vi "运维调试_氨氮.vi"() -> ()   [LabVIEW 2016, in "斯坦道氨氮.lvlib"]
uses:
  <vilib>/Utility/miscctls.llb/LVPointTypeDef.ctl
  <vilib>/Utility/config.llb/NI_LVConfig.lvlib
  <vilib>/ptbypt/NI_PtbyPt.lvlib
panel:
  in  "仪器参数设置":bool
  in  "模块启用":bool
  in  "串口设置":bool
  in  "备用系数一键写入":bool
  in  "公式一键写入":bool
  in  "流程路径":path=path "C:/Users/STD/Documents/斯坦道流程文件/流程.xml"
  in  "曲线模型":cluster{"X^2":dbl, "X":dbl, "B":dbl, "r^2":dbl}(xcontrol)
  out "字符串":string
  in  "质控参数设置":bool
  in  "自动测试量程配置":T1
  out "温度2":sgl
  out "温度1":sgl
  out "ADC":sgl
  out "固件版本号":string
  in  "数组":string[](array[string])
  in  "备用系数写入":bool
  in  "备用系数读取":bool
  in  "备用系数":T2
  in  "量程切换阈值写入":bool
  in  "量程切换阈值读取":bool
  in  "量程切换阈值":cluster{"阈值":dbl, "标液浓度":dbl}
  in  "参数下拉列表":enum16{"总磷", "总氮", "氨氮"}(ring)=enum."氨氮"
  in  "量程下拉列表":enum16{"低量程", "高量程"}(ring)
  in  "测量模式下拉列表":enum16{"水样测量", "零点核查", "跨度核查", "标样核查", "加标回收"}(ring)
  in  "公式":cluster{"X^2":dbl, "X":dbl, "b":dbl}
  in  "写公式":bool
  in  "读公式":bool
  in  "返回":bool
  in  "设置":bool
  out "序列号":string="序列号"
  out "测量数据":T3(xcontrol)
  out "集成报警信息":string
  out "定时启动":bool
  out "运行状态":T4(xcontrol)
  in  "停止":bool
  in  "手动启动":bool
  in  "单步测试":bool
  in  "总磷氨氮调试":u16[](xcontrol)
  out "F3":sgl format="%#.6f"
  out "F2":sgl format="%#.6f"
  out "F1":sgl format="%#.6f"
  out "F0":sgl format="%#.6f"
  out "多列列表框":i32(listbox)
  # "参数设置"
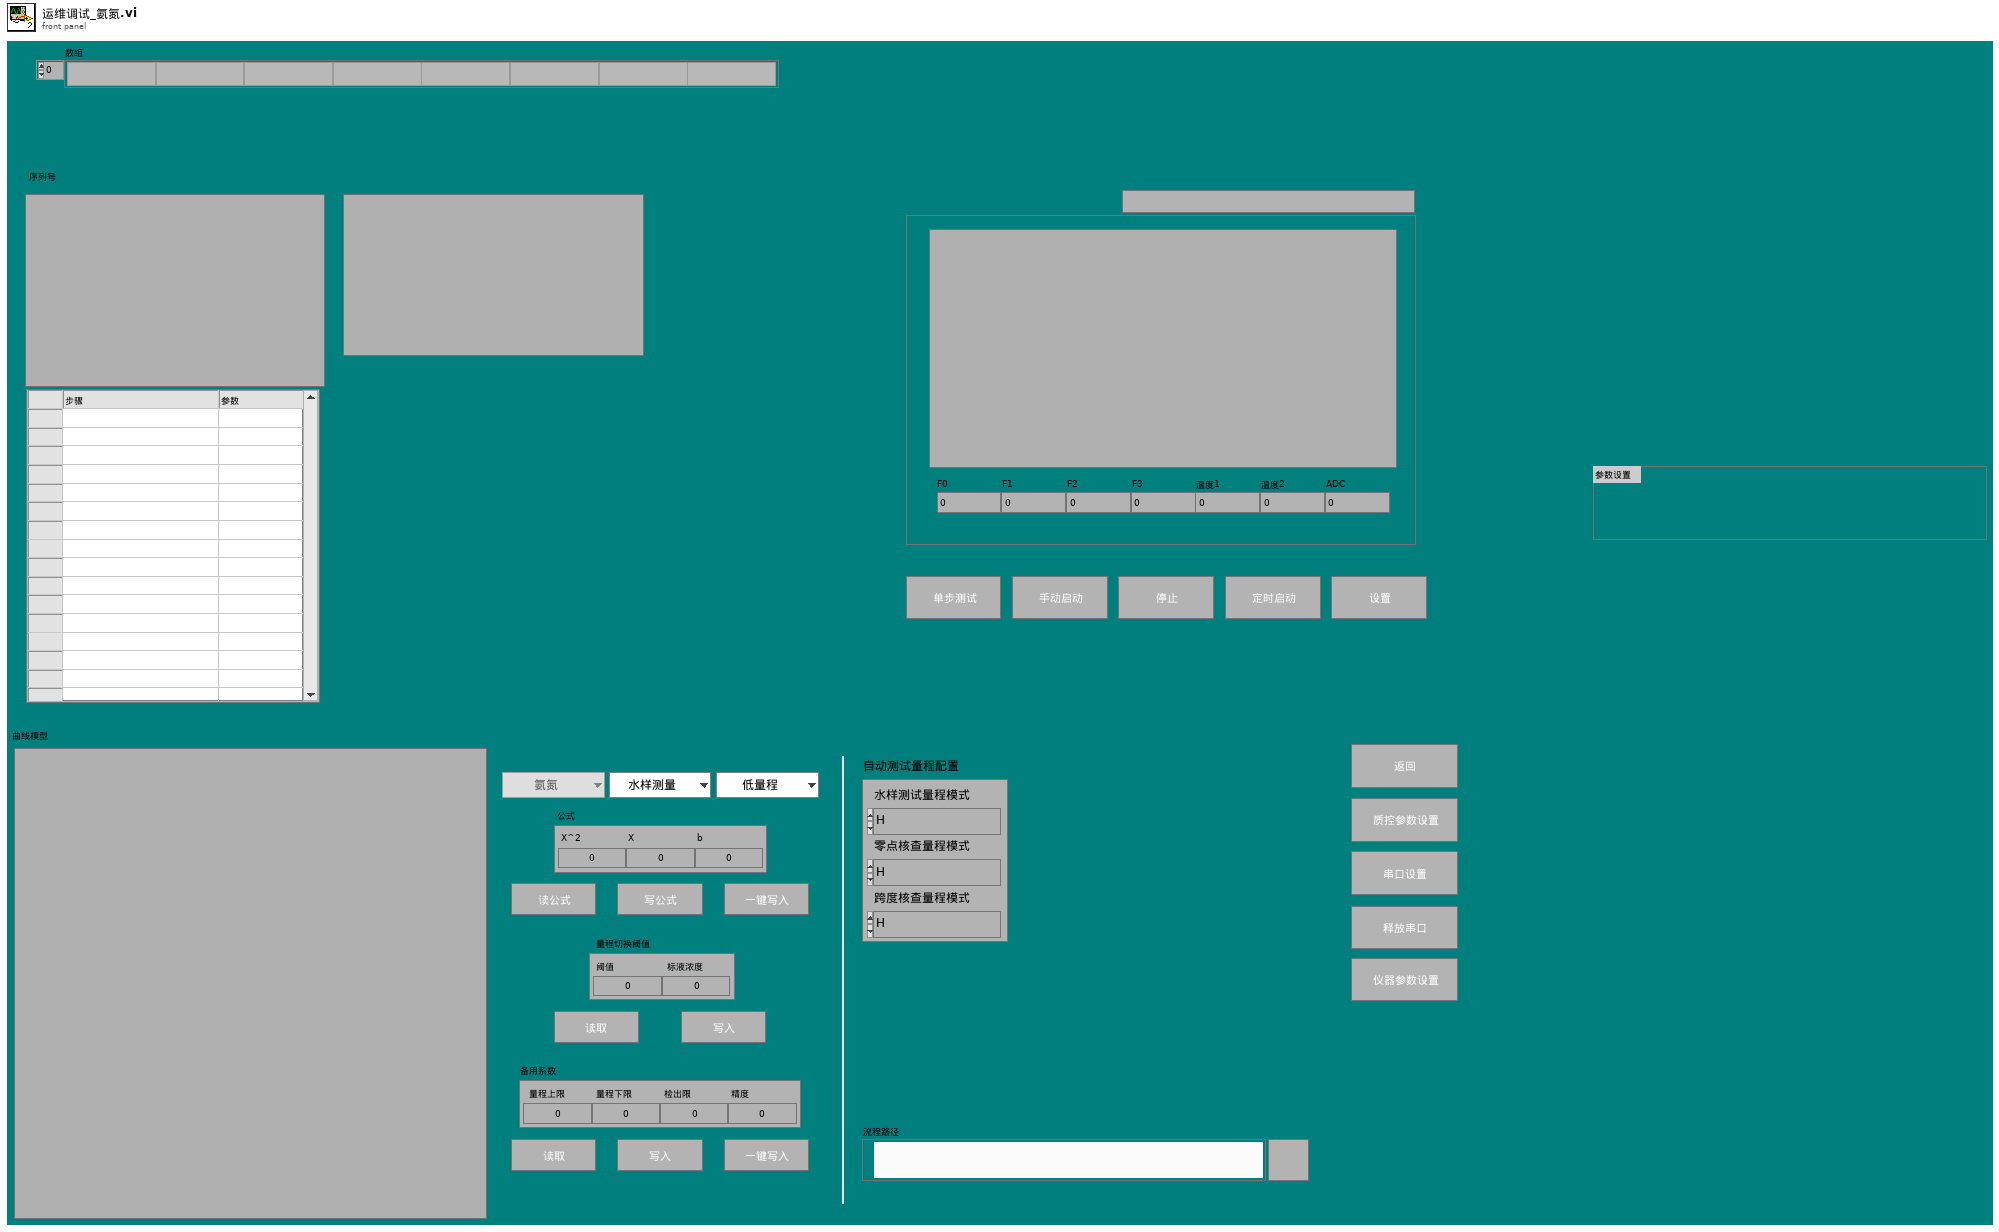
[diagram p1: front panel]
types:
  T1 = cluster{"水样测试量程模式":enum16{"H", "L", "AUTO"}, "空白核查量程模式":enum16{"H", "L", "AUTO"}, "跨度核查量程模式":enum16{"H", "L", "AUTO"}}
  T2 = cluster{"量程上限":dbl, "量程下限":dbl, "检出限":dbl, "精度":dbl}
  T3 = cluster{"flowid":u16, "测量精度":u16, "测量数据区":cluster{"因子编码":u32, "单位":u16, "标样参考值":sgl, "水样数据时间":timestamp, "水样实测值":sgl, "水样数据标识":string, "标样数据时间":timestamp, "标样实测值":sgl, "标样数据标识":string, "空白数据时间":timestamp, "空白实测值":sgl, "空白数据标识":string, "零点核查数据时间":timestamp, "零点核查实测值":sgl, "零点核查数据标识":string, "跨度核查数据时间":timestamp, "跨度核查实测值":sgl, "跨度核查数据标识":string, "加标回收数据时间":timestamp, "加标回收实测值":sgl, "加标回收数据标识":string, "平行样数据时间":timestamp, "平行样实测值":sgl, "平行样数据标识":string, "F0":sgl, "F1":sgl, "F2":sgl, "F3":sgl, "F4":sgl, "F5":sgl, "F6":sgl, "F7":sgl, "温度":sgl, "湿度":sgl, "X值":sgl}}
  T4 = cluster{"系统时间":timestamp, "工作状态":enum16{"空闲", "水样测试", "标样核查", "零点核查", "跨度核查", "空白测试", "平行样测试", "加标回收", "空白校准", "标样校准", "初始化（清洗）"}, "测量模式":enum16{"待机", "连续模式", "周期模式", "定点模式", "受控模式", "手动模式"}, "告警代码":u16, "故障代码":u16, "日志代码":u16, "软件版本":u16, "F0":sgl, "F1":sgl, "F2":sgl, "F3":sgl, "T":sgl, "H":sgl, "id":u16, "flowid":u16, "量程":u16, "总磷控温温度1":sgl, "营养盐控温温度2":sgl, "ADC":sgl}
  T5 = enum16{"启动测量", "标样核查", "零点核查", "跨度核查", "空白测试", "平行样测试", "加标回收", "空白校准", "标样校准", "初始化（清洗）", "停止测试", "仪器重启", "校时", "模式设置", "测量间隔设置"}
  T6 = cluster{"控制命令":enum16{"启动测量", "标样核查", "零点核查", "跨度核查", "空白测试", "平行样测试", "加标回收", "空白校准", "标样校准", "初始化（清洗）", "停止测试", "仪器重启", "校时", "模式设置", "测量间隔设置"}, "周期设置类型":enum16{"定点启动", "间隔启动"}, "定时功能启用":bool, "定时间隔":dbl, "24H周期设置":bool[], "零点核查时间":u16, "跨度核查时间":u16, "质控频次":enum16{"关闭", "每天", "星期一", "星期二", "星期三", "星期四", "星期五", "星期六", "星期日"}}
  T7 = enum16{"关闭", "每天", "星期一", "星期二", "星期三", "星期四", "星期五", "星期六", "星期日"}
  T8 = typedef "LVDateTimeRec.ctl" = cluster{"秒数的小数部分":dbl, "秒":i32, "分":i32, "时":i32, "日":i32, "月":i32, "年":i32, "天数（周）":i32, "天数（年）":i32, "DST":i32}
  T9 = enum16{"空闲", "水样测试", "标样核查", "零点核查", "跨度核查", "空白测试", "平行样测试", "加标回收", "空白校准", "标样校准", "初始化（清洗）"}
  T10 = enum32{"Bad", "Idle", "Run top level", "Running"}
  T11 = typedef "LVPointTypeDef.ctl" = cluster{"Horizontal":i16, "Vertical":i16}
  T12 = cluster{"因子编码":u32, "单位":u16, "标样参考值":sgl, "水样数据时间":timestamp, "水样实测值":sgl, "水样数据标识":string, "标样数据时间":timestamp, "标样实测值":sgl, "标样数据标识":string, "空白数据时间":timestamp, "空白实测值":sgl, "空白数据标识":string, "零点核查数据时间":timestamp, "零点核查实测值":sgl, "零点核查数据标识":string, "跨度核查数据时间":timestamp, "跨度核查实测值":sgl, "跨度核查数据标识":string, "加标回收数据时间":timestamp, "加标回收实测值":sgl, "加标回收数据标识":string, "平行样数据时间":timestamp, "平行样实测值":sgl, "平行样数据标识":string, "F0":sgl, "F1":sgl, "F2":sgl, "F3":sgl, "F4":sgl, "F5":sgl, "F6":sgl, "F7":sgl, "温度":sgl, "湿度":sgl, "X值":sgl}
  T13 = typedef "NI_LVConfig.lvlib/Config Data RefNum.ctl" = refnum<k1>
  T14 = cluster{"参数下拉列表":enum16{"总磷", "总氮", "氨氮"}, "测量模式下拉列表":enum16{"水样测量", "零点核查", "跨度核查", "标样核查", "加标回收"}, "量程下拉列表":enum16{"低量程", "高量程"}}
  T15 = cluster{"启动模式":enum16{"跨度核查", "水样测量", "空白核查", "标样核查", "加标回收"}, "启动参数":u16, "量程":enum16{"低量程", "高量程"}}
  T16 = cluster{"时间标识":timestamp, "设备":string, "日志信息":string, "流程参数":string}
  T17 = cluster{"时间标识":timestamp, "设备":string, "日志信息":string}
  T18 = typedef "LVRowAndColumnUnsignedTypeDef.ctl" = cluster{"Row":u32, "Column":u32}
  T19 = cluster{"站号":u16, "量程切换":enum32{"H", "L", "AUTO"}, "控制命令":enum16{"启动测量", "标样核查", "零点核查", "跨度核查", "空白测试", "平行样测试", "加标回收", "空白校准", "标样校准", "初始化（清洗）", "停止测试", "仪器重启", "校时", "模式设置", "测量间隔设置"}, "模式设置":enum16{"待机", "连续模式", "周期模式", "定点模式", "受控模式", "手动模式"}, "测量间隔":u16}
  T20 = cluster{"氨氮跨度值":dbl, "氨氮零点标准液浓度":dbl, "氨氮跨度标准液浓度":dbl, "氨氮标准液标准浓度":dbl}
  T21 = cluster{"确定":bool, "跨度值":dbl, "零点标准液浓度":dbl, "跨度标准液浓度":dbl, "标准液标准浓度":dbl}
  T22 = cluster{"测量量程":dbl, "测量精度":dbl, "测量间隔":dbl, "消解温度":dbl, "消解时长":dbl, "空白校准时间":timestamp, "曲线截距":dbl, "曲线斜率":dbl, "测量检出限":dbl, "测量信号值":dbl, "线性相关系数":dbl, "二次多项式系数":dbl, "标样校准时间":timestamp, "稀释倍数":dbl, "三项式系数":dbl, "空白标定系数":dbl, "量程系数":dbl, "F0/ORPA":dbl, "F1/ORPB":dbl, "F2/ORPK":dbl, "F3":dbl, "F4":dbl, "F5":dbl, "F6":dbl, "F7":dbl, "X0/滴定数":dbl, "量程":dbl}
  T23 = cluster{"确定":bool, "测量量程":dbl, "测量精度":dbl, "测量间隔":dbl, "消解温度":dbl, "消解时长":dbl, "空白校准时间":timestamp, "曲线截距":dbl, "曲线斜率":dbl, "测量检出限":dbl, "测量信号值":dbl, "线性相关系数":dbl, "二次多项式系数":dbl, "标样校准时间":timestamp, "稀释倍数":dbl, "三项式系数":dbl, "空白标定系数":dbl, "量程系数":dbl, "F0/ORPA":dbl, "F1/ORPB":dbl, "F2/ORPK":dbl, "F3":dbl, "F4":dbl, "F5":dbl, "F6":dbl, "F7":dbl, "X0/滴定数":dbl, "量程":dbl}
  T24 = cluster{"控制命令":enum16{"启动测量", "标样核查", "零点核查", "跨度核查", "空白测试", "平行样测试", "加标回收", "空白校准", "标样校准", "初始化（清洗）", "停止测试", "仪器重启", "校时", "模式设置", "测量间隔设置"}, "周期设置类型":enum16{"定点启动", "间隔启动"}, "定时功能启用":bool, "定时间隔":dbl, "24H周期设置":bool[], "空白核查时间":u16, "跨度核查时间":u16, "质控频次":enum16{"关闭", "每天", "星期一", "星期二", "星期三", "星期四", "星期五", "星期六", "星期日"}}
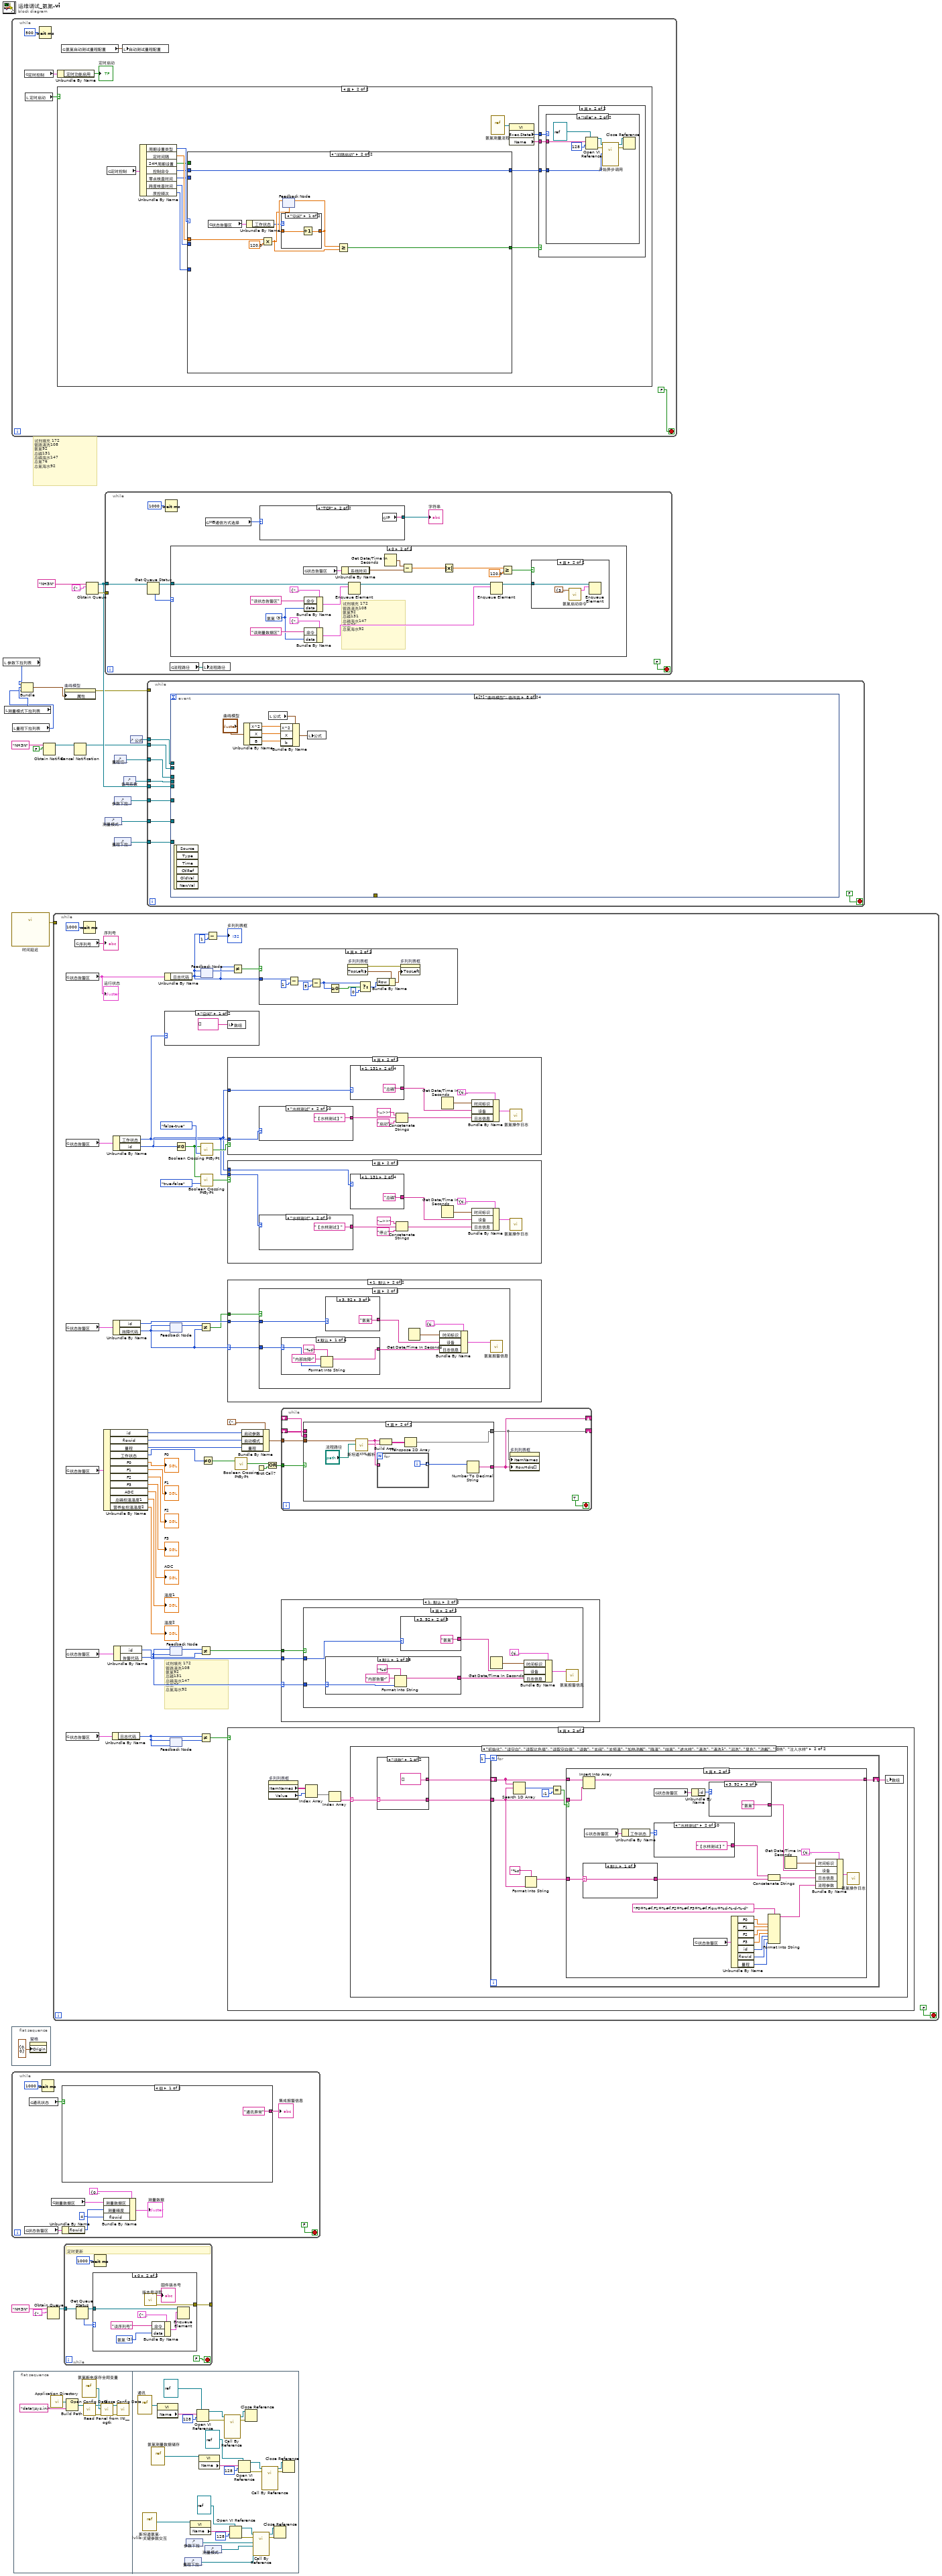
[diagram p0: block diagram]
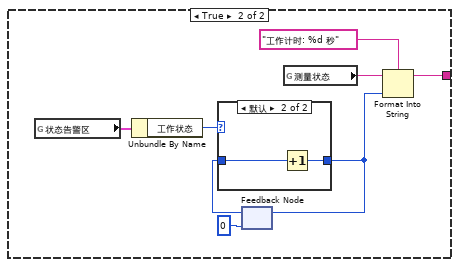
[diagram p3: hidden frame]
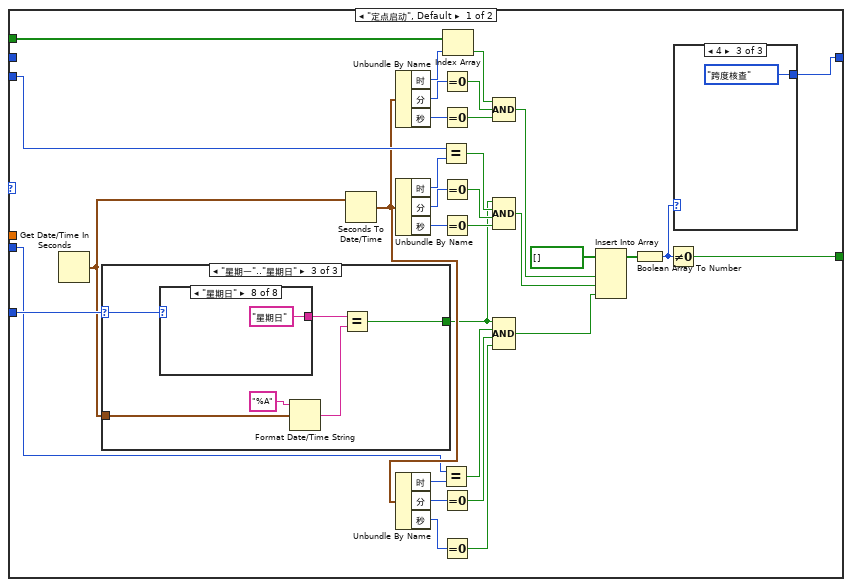
[diagram p8: hidden frame]
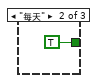
[diagram p10: hidden frame]
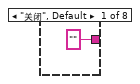
[diagram p11: hidden frame]
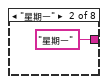
[diagram p12: hidden frame]
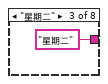
[diagram p13: hidden frame]
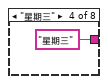
[diagram p14: hidden frame]
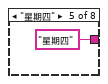
[diagram p15: hidden frame]
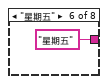
[diagram p16: hidden frame]
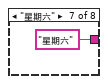
[diagram p17: hidden frame]
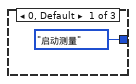
[diagram p18: hidden frame]
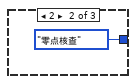
[diagram p19: hidden frame]
diagram:
  # "试剂填充 172 \n管路清洗108\n氨氮92\n总磷131\n总磷海水147\n总氮76\n总氮海水92"
  n1 = local read "参数下拉列表"() -> (w4:enum16{"总磷", "总氮", "氨氮"})
  n2 = local read "测量模式下拉列表"() -> (w3:enum16{"水样测量", "零点核查", "跨度核查", "标样核查", "加标回收"})
  n3 = while {
    stop <- FALSE stop-if-true
    n4 = global read "氨氮断电保存全局变量.vi" "定时控制"() -> (w25:T6)
    n5 = local read "定时启动"() -> (w27:bool)
    n6 = Wait (ms)(milliseconds to wait=u32 500 ("等待时间（毫秒）")) -> ()  [unwired: 1 out]
    n7 = Unbundle By Name(w25) -> ("定时功能启用"=→"定时启动":bool)
    n8 = case shown="真" w27 {
      frame False {
      }
      frame True {
        n9 = global read "氨氮断电保存全局变量.vi" "定时控制"() -> (w42:T6)
        n10 = Unbundle By Name(w42) -> ("周期设置类型"=w41:enum16{"定点启动", "间隔启动"}, "定时间隔"=w40:dbl, "24H周期设置"=w39:bool[], "控制命令"=w34:T5, "零点核查时间"=w32:u16, "跨度核查时间"=w31:u16, "质控频次"=w30:T7)
        n11 = case shown="\"间隔启动\"" w41 {
          tunnel: w40 -> [_ w111]
          tunnel: w39 -> [w77 _]
          tunnel: [w55 w109] -> w38
          tunnel: w34 -> [_ w107]
          tunnel: [w81 w107] -> w33
          tunnel: w30 -> [w80 _]
          tunnel: w32 -> [w73 _]
          tunnel: w31 -> [w62 _]
          frame "定点启动", Default {
            n12 = Get Date/Time In Seconds() -> (seconds since 1Jan1904=w79:timestamp)
            n13 = case shown="\"星期一\"..\"星期日\"" w80 {
              selector: w80 -> [_ _ w91]
              tunnel: w79 -> [_ _ w92]
              tunnel: [_ TRUE w88] -> w61
              frame "关闭", Default {
              }
              frame "每天" {
              }
              frame "星期一".."星期日" {
                n14 = case shown="\"星期日\"" w91 {
                  tunnel: ["" ("时间格式字符串(%c)") "星期一" ("时间格式字符串(%c)") "星期二" ("时间格式字符串(%c)") "星期三" ("时间格式字符串(%c)") "星期四" ("时间格式字符串(%c)") "星期五" ("时间格式字符串(%c)") "星期六" ("时间格式字符串(%c)") "星期日" ("时间格式字符串(%c)")] -> w90
                  frame "关闭", Default {
                  }
                  frame "星期一" {
                  }
                  frame "星期二" {
                  }
                  frame "星期三" {
                  }
                  frame "星期四" {
                  }
                  frame "星期五" {
                  }
                  frame "星期六" {
                  }
                  frame "星期日" {
                  }
                }
                n15 = Format Date/Time String(time format string (%c)="%A" ("时间格式字符串(%c)"), seconds (now)=w92) -> (date/time string=w89:string)  [unwired: 1 in]
                n16 = Equal?(x=w90, y=w89) -> (x = y?=w88:bool)
              }
            }
            n17 = Seconds To Date/Time(time stamp (now)=w79) -> (date time rec=w63:T8)  [unwired: 1 in]
            n18 = Unbundle By Name(w63) -> ("时"=w86:i32, "分"=w84:i32, "秒"=w85:i32)
            n19 = Unbundle By Name(w63) -> ("时"=w74:i32, "分"=w76:i32, "秒"=w75:i32)
            n20 = Unbundle By Name(w63) -> ("时"=w66:i32, "分"=w64:i32, "秒"=w65:i32)
            n21 = Equal?(x=w73, y=w74) -> (x = y?=w72:bool)
            n22 = Equal?(x=w62, y=w66) -> (x = y?=w67:bool)
            n23 = Equal To 0?(x=w84) -> (x = 0?=w83:bool)
            n24 = Equal To 0?(x=w85) -> (x = 0?=w82:bool)
            n25 = Equal To 0?(x=w76) -> (x = 0?=w71:bool)
            n26 = Equal To 0?(x=w75) -> (x = 0?=w70:bool)
            n27 = Equal To 0?(x=w64) -> (x = 0?=w68:bool)
            n28 = Equal To 0?(x=w65) -> (x = 0?=w69:bool)
            n29 = Index Array(array=w77, index=w86) -> (element=w78:bool)
            n30 = Compound Arithmetic op=AND ("复合运算")(w78, w83, w82) -> (w59:bool)
            n31 = Compound Arithmetic op=AND ("复合运算")(w61, w72, w71, w70) -> (w58:bool)
            n32 = Compound Arithmetic op=AND ("复合运算")(w61, w67, w68, w69) -> (w57:bool)
            n33 = Insert Into Array(array=bool[] [], new element #1=w59, new element #2=w58, new element #3=w57) -> (w56:bool[])  [unwired: 1 in]
            n34 = Boolean Array To Number(Boolean array=w56) -> (number=w54:u32)
            n35 = Not Equal To 0?(x=w54) -> (x != 0?=w55:bool)
            n36 = case shown="4" w54 {
              tunnel: [T5."启动测量" ("控制命令") T5."零点核查" ("控制命令") T5."跨度核查" ("控制命令")] -> w81
              frame 0, Default {
              }
              frame 2 {
              }
              frame 4 {
              }
            }
          }
          frame "间隔启动" {
            n37 = global read "VAR氨氮全局变量.vi" "状态告警区"() -> (w106:T4)
            n38 = Unbundle By Name(w106) -> ("工作状态"=w105:T9)
            n39 = Multiply(x=w111, y=120.0) -> (x*y=w108:dbl)
            n40 = feedback #1(w108) -> (w113:dbl)
            n41 = case shown="\"空闲\"" w105 {
              tunnel: w113 -> [w115 _]
              tunnel: [w114 _] -> w112
              frame "空闲" {
                n42 = Increment(x=w115) -> (x+1=w114:dbl)
              }
              frame "水样测试", Default {
              }
            }
            n43 = feedback-in #1(w112) -> ()
            n44 = Greater Or Equal?(x=w112, y=w108) -> (x >= y?=w109:bool)
          }
        }
        n45 = vi-ref "氨氮测量流程.vi"() -> (w37:refnum<vi>)
        n46 = property class="VI"(reference=w37) -> ("Exec.State"=w36:T10, "Name"=w35:string)  [unwired: 1 in, 2 out]
        n47 = case shown="真" w38 {
          tunnel: w35 -> [_ w45]
          tunnel: w33 -> [_ w44]
          tunnel: w36 -> [_ w43]
          frame False {
          }
          frame True {
            n48 = case shown="\"Idle\"" w43 {
              tunnel: w45 -> [_ w49]
              tunnel: w44 -> [_ w47]
              frame "Bad", Default {
              }
              frame "Idle" {
                n49 = Open VI Reference(type specifier VI Refnum (for type only)=refnum<vi> refnum, vi path=w49, options=128 ("选项")) -> (vi reference=w50:refnum<vi>, error out=w51:errorcluster)  [unwired: 3 in]
                n50 = call-by-ref "开始异步调用"(reference=w50, error in=w51, "控制命令"=w47) -> (reference out=w52:refnum<vi>, error out=w53:errorcluster)  [unwired: 11 in]
                n51 = Close Reference(reference=w52, error in (no error)=w53) -> ()  [unwired: 1 out]
              }
            }
          }
        }
      }
    }
    n52 = global read "氨氮断电保存全局变量.vi" "氨氮自动测试量程配置"() -> (w26:T1)
    n53 = local write "自动测试量程配置"(w26) -> ()
  }
  n54 = call "时间延迟"() -> ("error out"=w13:errorcluster)  [unwired: 11 in]
  n55 = flat-sequence {
    frame #0 {
      n56 = property on="窗格" class="Pane"("Origin"=T11 {"Horizontal"=0, "Vertical"=0} ("原点")) -> ()  [unwired: 2 in, 2 out]
    }
  }
  n57 = while {
    stop <- FALSE stop-if-true
    n58 = global read "VAR氨氮全局变量.vi" "状态告警区"() -> (w122:T4)
    n59 = global read "VAR氨氮全局变量.vi" "通讯状态"() -> (w124:bool)
    n60 = Wait (ms)(milliseconds to wait=u32 1000 ("等待时间（毫秒）")) -> ()  [unwired: 1 out]
    n61 = global read "VAR氨氮全局变量.vi" "测量数据区"() -> (w117:T12)
    n62 = case shown="假" w124 {
      tunnel: ["通讯异常" ("集成报警信息") w129] -> w123
      frame False {
      }
      frame True {
        n63 = global read "VAR氨氮全局变量.vi" "状态告警区"() -> (w135:T4)
        n64 = Unbundle By Name(w135) -> ("工作状态"=w134:T9)
        n65 = feedback #2(0) -> (w132:i32)
        n66 = case shown="默认" w134 {
          tunnel: w132 -> [_ w137]
          tunnel: [_ w136] -> w130
          frame "空闲" {
          }
          frame Default {
            n67 = Increment(x=w137) -> (x+1=w136:i32)
          }
        }
        n68 = feedback-in #2(w130) -> ()
        n69 = global read "VAR氨氮全局变量.vi" "测量状态"() -> (w128:string)
        n70 = Format Into String(format string="工作计时: %d 秒" ("格式字符串"), initial string=w128, w130) -> (resulting string=w129:string)  [unwired: 1 in, 1 out]
      }
    }
    "集成报警信息" <- w123
    n71 = Unbundle By Name(w122) -> ("flowid"=w121:u16)
    n72 = Bundle By Name(cluster=T3 {"flowid"=0, "测量精度"=0, "测量数据区"={"因子编码"=0, "单位"=0, "标样参考值"=0.0, "水样数据时间"=timestamp(0 s since 1904-01-01), "水样实测值"=0.0, "水样数据标识"="", "标样数据时间"=timestamp(0 s since 1904-01-01), "标样实测值"=0.0, "标样数据标识"="", "空白数据时间"=timestamp(0 s since 1904-01-01), "空白实测值"=0.0, "空白数据标识"="", "零点核查数据时间"=timestamp(0 s since 1904-01-01), "零点核查实测值"=0.0, "零点核查数据标识"="", "跨度核查数据时间"=timestamp(0 s since 1904-01-01), "跨度核查实测值"=0.0, "跨度核查数据标识"="", "加标回收数据时间"=timestamp(0 s since 1904-01-01), "加标回收实测值"=0.0, "加标回收数据标识"="", "平行样数据时间"=timestamp(0 s since 1904-01-01), "平行样实测值"=0.0, "平行样数据标识"="", "F0"=0.0, "F1"=0.0, "F2"=0.0, "F3"=0.0, "F4"=0.0, "F5"=0.0, "F6"=0.0, "F7"=0.0, "温度"=0.0, "湿度"=0.0, "X值"=0.0}} ("总氮测量数据"), "测量数据区"=w117, "测量精度"=u16 4, "flowid"=w121) -> (→"测量数据":T3)
  }
  n73 = local read "量程下拉列表"() -> (w2:enum16{"低量程", "高量程"})
  n74 = flat-sequence {
    frame #0 {
      n75 = call <vilib>:"Application Directory.vi"() -> ("Application Directory"=w145:path)
      n76 = Build Path(base path=w145, name or relative path="data\\sys.ini" ("名称或相对路径")) -> (appended path=w143:path)
      n77 = vi-ref "氨氮断电保存全局变量.vi"() -> (w141:refnum<vi>)
      n78 = call <vilib>:"Open Config Data.vi"("configuration file path"=w143) -> ("error out"=w139:errorcluster, "refnum"=w142:T13)  [unwired: 8 in, 1 out]
      n79 = call <userlib>:"Read Panel from INI__ogtk.vi"("error in (no error)"=w139, "VI ref"=w141, "refnum"=w142) -> ("error out"=w138:errorcluster, "refnum out"=w140:T13)  [unwired: 7 in]
      n80 = call <vilib>:"Close Config Data.vi"("error in (no error)"=w138, "refnum"=w140) -> ()  [unwired: 8 in, 2 out]
    }
    frame #1 {
      n81 = vi-ref "通讯.vi"() -> (w172:refnum<vi>)
      n82 = vi-ref "斯坦道氨氮.lvlib:关键参数交互.vi"() -> (w149:refnum<vi>)
      n83 = vi-ref "氨氮测量数据储存.vi"() -> (w164:refnum<vi>)
      n84 = property class="VI"(reference=w172) -> ("Name"=w171:string)  [unwired: 1 in, 2 out]
      n85 = control-ref of="量程下拉列表"() -> (w146:refnum<vi>)
      n86 = control-ref of="参数下拉列表"() -> (w148:refnum<vi>)
      n87 = property class="VI"(reference=w149) -> ("Name"=w156:string)  [unwired: 1 in, 2 out]
      n88 = Open VI Reference(type specifier VI Refnum (for type only)=refnum<vi> refnum, vi path=w171, options=128 ("选项")) -> (vi reference=w169:refnum<vi>, error out=w167:errorcluster)  [unwired: 3 in]
      n89 = property class="VI"(reference=w164) -> ("Name"=w157:string)  [unwired: 1 in, 2 out]
      n90 = control-ref of="测量模式下拉列表"() -> (w147:refnum<vi>)
      n91 = call-by-ref "?"(reference=w169, error in=w167) -> (reference out=w165:refnum<vi>, error out=w166:errorcluster)  [unwired: 12 in]
      n92 = Open VI Reference(type specifier VI Refnum (for type only)=refnum<vi> refnum, vi path=w156, options=128 ("选项")) -> (vi reference=w154:refnum<vi>, error out=w152:errorcluster)  [unwired: 3 in]
      n93 = Open VI Reference(type specifier VI Refnum (for type only)=refnum<vi> refnum, vi path=w157, options=128 ("选项")) -> (vi reference=w159:refnum<vi>, error out=w161:errorcluster)  [unwired: 3 in]
      n94 = Close Reference(reference=w165, error in (no error)=w166) -> ()  [unwired: 1 out]
      n95 = call-by-ref "?"(reference=w154, error in=w152, "量程下拉列表"=w146, "测量模式下拉列表"=w147, "参数下拉列表"=w148) -> (reference out=w150:refnum<vi>, error out=w151:errorcluster)  [unwired: 9 in]
      n96 = call-by-ref "?"(reference=w159, error in=w161) -> (reference out=w163:refnum<vi>, error out=w162:errorcluster)  [unwired: 12 in]
      n97 = Close Reference(reference=w150, error in (no error)=w151) -> ()  [unwired: 1 out]
      n98 = Close Reference(reference=w163, error in (no error)=w162) -> ()  [unwired: 1 out]
    }
  }
  n99 = Bundle("参数下拉列表"=w4, "测量模式下拉列表"=w3, "量程下拉列表"=w2) -> (w1:T14)  [unwired: 1 in]
  n100 = Obtain Notifier(name (unnamed)="NH3N" ("名称（未命名）"), notification data type=FALSE) -> (notifier out=w6:refnum<notifier>)  [unwired: 2 in, 2 out]
  n101 = Obtain Queue(name (unnamed)="NH3N" ("名称（未命名）"), element data type=cluster{"命令":string, "data":variant} {"命令"="", "data"=variant}) -> (queue out=w10:refnum<queue>)  [unwired: 3 in, 2 out]
  n102 = while {
    tunnel: w13 -> [_]
    stop <- FALSE stop-if-true
    # "试剂填充 172 \n管路清洗108\n氨氮92\n总磷131\n总磷海水147\n总氮76\n总氮海水92"
    n103 = global read "VAR氨氮全局变量.vi" "状态告警区"() -> (w206:T4)
    "运行状态" <- w206
    n104 = global read "VAR氨氮全局变量.vi" "状态告警区"() -> (w193:T4)
    n105 = global read "VAR氨氮全局变量.vi" "状态告警区"() -> (w198:T4)
    n106 = global read "VAR氨氮全局变量.vi" "状态告警区"() -> (w214:T4)
    n107 = global read "VAR氨氮全局变量.vi" "状态告警区"() -> (w203:T4)
    n108 = global read "VAR氨氮全局变量.vi" "状态告警区"() -> (w191:T4)
    n109 = global read "VAR氨氮全局变量.vi" "序列号"() -> (→"序列号":string)
    n110 = Wait (ms)(milliseconds to wait=u32 1000 ("等待时间（毫秒）")) -> ()  [unwired: 1 out]
    n111 = Unbundle By Name(w214) -> ("id"=w211:u16, "flowid"=w213:u16, "量程"=w212:u16, "工作状态"=w181:T9, "F0"=→"F0":sgl, "F1"=→"F1":sgl, "F2"=→"F2":sgl, "F3"=→"F3":sgl, "ADC"=→"ADC":sgl, "总磷控温温度1"=→"温度1":sgl, "营养盐控温温度2"=→"温度2":sgl)
    n112 = Unbundle By Name(w191) -> ("日志代码"=w190:u16)
    n113 = Unbundle By Name(w193) -> ("工作状态"=w177:T9, "id"=w176:u16)
    n114 = Unbundle By Name(w198) -> ("id"=w197:u16, "故障代码"=w194:u16)
    n115 = Unbundle By Name(w203) -> ("id"=w202:u16, "告警代码"=w199:u16)
    n116 = Unbundle By Name(w206) -> ("日志代码"=w187:u16)
    n117 = case shown="\"空闲\"" w177 {
      frame "空闲" {
        n118 = local write "数组"(string[] [] ("数组")) -> ()
      }
      frame "水样测试", Default {
      }
    }
    n119 = feedback #3(w194) -> (w195:u16)
    n120 = feedback-in #3(w194) -> ()
    n121 = feedback #4(w199) -> (w200:u16)
    n122 = feedback-in #4(w199) -> ()
    n123 = feedback #5(w190) -> (w192:u16)
    n124 = feedback-in #5(w190) -> ()
    n125 = Not Equal To 0?(x=w176) -> (x != 0?=w174:bool)
    n126 = Not Equal?(x=w195, y=w194) -> (x != y?=w196:bool)
    n127 = Not Equal?(x=w200, y=w199) -> (x != y?=w201:bool)
    n128 = Not Equal?(x=w190, y=w192) -> (x != y?=w189:bool)
    n129 = feedback-in #6(w187) -> ()
    n130 = feedback #6(w187) -> (w219:u16)
    n131 = call <vilib>:"Boolean Crossing PtByPt.vi"("direction"=enum16{"either", "false-true", "true-false"}."false-true", "input"=w174) -> ("crossing"=w178:bool)  [unwired: 1 in]
    n132 = call <vilib>:"Boolean Crossing PtByPt.vi"("direction"=enum16{"either", "false-true", "true-false"}."true-false", "input"=w174) -> ("crossing"=w173:bool)  [unwired: 1 in]
    n133 = Not Equal To 0?(x=w181) -> (x != 0?=w216:bool)
    n134 = Subtract(x=w187, y=1) -> (x-y=→"多列列表框":i32)
    n135 = case shown="真" w178 {
      tunnel: w176 -> [_ w246]
      tunnel: w177 -> [_ w245]
      frame False {
      }
      frame True {
        n136 = case shown="\"水样测试\"" w245 {
          tunnel: [_ "【水样测试】" ("字符串") "【标样核查】" ("字符串") "【零点核查】" ("字符串") "【跨度核查】" ("字符串") "【空白测试】" ("字符串") "【平行样测试】" ("字符串") "【加标回收】" ("字符串") "【空白校准】" ("字符串") "【标样校准】" ("字符串")] -> w250
          frame "空闲", Default {
          }
          frame "水样测试" {
          }
          frame "标样核查" {
          }
          frame "零点核查" {
          }
          frame "跨度核查" {
          }
          frame "空白测试" {
          }
          frame "平行样测试" {
          }
          frame "加标回收" {
          }
          frame "空白校准" {
          }
          frame "标样校准" {
          }
        }
        n137 = case shown="1, 131" w246 {
          tunnel: [_ "总磷" ("table输入") "氨氮" ("table输入") "总氮" ("table输入")] -> w251
          frame Default {
          }
          frame 1, 131 {
          }
          frame 3, 92 {
          }
          frame 2, 76 {
          }
        }
        n138 = Concatenate Strings("-->>" ("字符串"), w250, "启动" ("字符串")) -> (w249:string)
        n139 = Get Date/Time In Seconds() -> (seconds since 1Jan1904=w252:timestamp)
        n140 = Bundle By Name(cluster=T16 {"时间标识"=timestamp(0 s since 1904-01-01), "设备"="", "日志信息"="", "流程参数"=""} ("data in"), "时间标识"=w252, "设备"=w251, "日志信息"=w249) -> (w244:T16)
        n141 = call "氨氮操作日志.vi"("data in"=w244) -> ()  [unwired: 11 in]
      }
    }
    n142 = case shown="真" w173 {
      tunnel: w176 -> [_ w224]
      tunnel: w177 -> [_ w223]
      frame False {
      }
      frame True {
        n143 = case shown="\"水样测试\"" w223 {
          tunnel: [_ "【水样测试】" ("字符串") "【标样核查】" ("字符串") "【零点核查】" ("字符串") "【跨度核查】" ("字符串") "【空白测试】" ("字符串") "【平行样测试】" ("字符串") "【加标回收】" ("字符串") "【空白校准】" ("字符串") "【标样校准】" ("字符串")] -> w228
          frame "空闲", Default {
          }
          frame "水样测试" {
          }
          frame "标样核查" {
          }
          frame "零点核查" {
          }
          frame "跨度核查" {
          }
          frame "空白测试" {
          }
          frame "平行样测试" {
          }
          frame "加标回收" {
          }
          frame "空白校准" {
          }
          frame "标样校准" {
          }
        }
        n144 = case shown="1, 131" w224 {
          tunnel: [_ "总磷" ("table输入") "氨氮" ("table输入") "总氮" ("table输入")] -> w229
          frame Default {
          }
          frame 1, 131 {
          }
          frame 3, 92 {
          }
          frame 2, 76 {
          }
        }
        n145 = Concatenate Strings("-->>" ("字符串"), w228, "停止" ("字符串")) -> (w227:string)
        n146 = Get Date/Time In Seconds() -> (seconds since 1Jan1904=w230:timestamp)
        n147 = Bundle By Name(cluster=T16 {"时间标识"=timestamp(0 s since 1904-01-01), "设备"="", "日志信息"="", "流程参数"=""} ("data in"), "时间标识"=w230, "设备"=w229, "日志信息"=w227) -> (w222:T16)
        n148 = call "氨氮操作日志.vi"("data in"=w222) -> ()  [unwired: 11 in]
      }
    }
    n149 = case shown="1, 默认" w194 {
      selector: w194 -> [_ w334]
      tunnel: w197 -> [_ w335]
      tunnel: w196 -> [_ w333]
      frame 0 {
      }
      frame 1, Default {
        n150 = case shown="真" w333 {
          tunnel: w335 -> [_ w342]
          tunnel: w334 -> [_ w337]
          frame False {
          }
          frame True {
            n151 = case shown="默认" w337 {
              selector: w337 -> [w344 _ _ _ _ _]
              tunnel: [w343 "无故障" "电机故障" "温度故障" "通讯故障" "滴定故障"] -> w336
              frame Default {
                n152 = Format Into String(format string="%d" ("格式字符串"), initial string="内部故障-" ("工作状态"), w344) -> (resulting string=w343:string)  [unwired: 1 in, 1 out]
              }
              frame 0 {
              }
              frame 1 {
              }
              frame 2 {
              }
              frame 3 {
              }
              frame 4 {
              }
            }
            n153 = case shown="3, 92" w342 {
              tunnel: [_ "总磷" ("table输入") "氨氮" ("table输入") "总氮" ("table输入")] -> w338
              frame Default {
              }
              frame 1, 131 {
              }
              frame 3, 92 {
              }
              frame 2, 76 {
              }
            }
            n154 = Get Date/Time In Seconds() -> (seconds since 1Jan1904=w339:timestamp)
            n155 = Bundle By Name(cluster=T17 {"时间标识"=timestamp(0 s since 1904-01-01), "设备"="", "日志信息"=""} ("data in"), "时间标识"=w339, "设备"=w338, "日志信息"=w336) -> (w340:T17)
            n156 = call "氨氮报警信息.vi"("data in"=w340) -> ()  [unwired: 10 in, 1 out]
          }
        }
      }
    }
    n157 = case shown="真" w189 {
      frame False {
      }
      frame True {
        n158 = property on="多列列表框" class="MCListbox (严格)"() -> ("ItemNames"=w269:string[][], "Value"=w270:i32)  [unwired: 2 in, 2 out]
        n159 = Index Array(array=w269, index (row)=w270) -> (element=w268:string[])  [unwired: 1 in]
        n160 = Index Array(array=w268) -> (element=w267:string)  [unwired: 1 in]
        n161 = case shown="\"初始化\", \"读空白\", \"读取比色值\", \"读取空白值\", \"读数\", \"关阀\", \"关恒温\", \"加热消解\", \"降温\", \"结束\", \"进水样\", \"清洗\", \"清洗1\", \"润洗\", \"显色\", \"消解\", \"预热\", \"注入水样\"" w267 {
          selector: w267 -> [_ w273]
          frame Default {
          }
          frame "初始化", "读空白", "读取比色值", "读取空白值", "读数", "关阀", "关恒温", "加热消解", "降温", "结束", "进水样", "清洗", "清洗1", "润洗", "显色", "消解", "预热", "注入水样" {
            n162 = case shown="\"读数\"" w273 {
              selector: w273 -> [w277 w279]
              tunnel: [w277 w279] -> w272
              tunnel: [string[] [] ("数组") "数组"] -> w271
              frame "读数" {
              }
              frame Default {
              }
            }
            n163 = for {
              N: 1 -> [_]
              tunnel: w272 -> [w281]
              shift-right: [w280] -> w274
              shift-left: w271 -> [w282]
              n164 = Search 1D Array(1D array=w282, element=w281) -> (index of element=w285:i32)  [unwired: 1 in]
              n165 = Format Into String(format string="%s" ("格式字符串"), w281) -> (resulting string=w286:string)  [unwired: 2 in, 1 out]
              n166 = Equal?(x=w285, y=-1) -> (x = y?=w283:bool)
              n167 = case shown="真" w283 {
                tunnel: w286 -> [_ w294]
                tunnel: w282 -> [w288 w298]
                tunnel: w281 -> [_ w297]
                tunnel: [w288 w296] -> w280
                frame False {
                }
                frame True {
                  n168 = Insert Into Array(array=w298, new element=w297) -> (w296:string[])  [unwired: 1 in]
                  n169 = case shown="默认" w294 {
                    selector: w294 -> [w323 w326 w329]
                    tunnel: [w323 w325 w328] -> w293
                    frame Default {
                    }
                    frame "初始化" {
                      n170 = Concatenate Strings("-->>" ("字符串"), w326) -> (w325:string)
                    }
                    frame "结束" {
                      n171 = Concatenate Strings("-->>" ("字符串"), w329) -> (w328:string)
                    }
                  }
                  n172 = global read "VAR氨氮全局变量.vi" "状态告警区"() -> (w292:T4)
                  n173 = Unbundle By Name(w292) -> ("工作状态"=w291:T9)
                  n174 = global read "VAR氨氮全局变量.vi" "状态告警区"() -> (w313:T4)
                  n175 = case shown="\"水样测试\"" w291 {
                    tunnel: [_ "【水样测试】" ("字符串") "【标样核查】" ("字符串") "【零点核查】" ("字符串") "【跨度核查】" ("字符串") "【空白测试】" ("字符串") "【平行样测试】" ("字符串") "【加标回收】" ("字符串") "【空白校准】" ("字符串") "【标样校准】" ("字符串")] -> w289
                    frame "空闲", Default {
                    }
                    frame "水样测试" {
                    }
                    frame "标样核查" {
                    }
                    frame "零点核查" {
                    }
                    frame "跨度核查" {
                    }
                    frame "空白测试" {
                    }
                    frame "平行样测试" {
                    }
                    frame "加标回收" {
                    }
                    frame "空白校准" {
                    }
                    frame "标样校准" {
                    }
                  }
                  n176 = Unbundle By Name(w313) -> ("id"=w312:u16)
                  n177 = global read "VAR氨氮全局变量.vi" "状态告警区"() -> (w308:T4)
                  n178 = case shown="3, 92" w312 {
                    tunnel: [_ "总磷" ("table输入") "氨氮" ("table输入") "总氮" ("table输入")] -> w310
                    frame Default {
                    }
                    frame 1, 131 {
                    }
                    frame 3, 92 {
                    }
                    frame 2, 76 {
                    }
                  }
                  n179 = Unbundle By Name(w308) -> ("F0"=w305:sgl, "F1"=w304:sgl, "F2"=w303:sgl, "F3"=w302:sgl, "id"=w301:u16, "flowid"=w300:u16, "量程"=w299:u16)
                  n180 = Concatenate Strings(w289, w293) -> (w290:string)
                  n181 = Format Into String(format string="F0=%#f,F1=%#f,F2=%#f,F3=%#f,Flow=%d-%-d-%-d" ("格式字符串"), w305, w304, w303, w302, w301, w300, w299) -> (resulting string=w306:string)  [unwired: 2 in, 1 out]
                  n182 = Get Date/Time In Seconds() -> (seconds since 1Jan1904=w309:timestamp)
                  n183 = Bundle By Name(cluster=T16 {"时间标识"=timestamp(0 s since 1904-01-01), "设备"="", "日志信息"="", "流程参数"=""} ("data in"), "时间标识"=w309, "设备"=w310, "日志信息"=w290, "流程参数"=w306) -> (w311:T16)
                  n184 = call "氨氮操作日志.vi"("data in"=w311) -> ()  [unwired: 11 in]
                }
              }
            }
            n185 = local write "数组"(w274) -> ()
          }
        }
      }
    }
    n186 = Not Equal?(x=w187, y=w219) -> (x != y?=w218:bool)
    n187 = call <vilib>:"Boolean Crossing PtByPt.vi"("input"=w216) -> ("crossing"=w180:bool)  [unwired: 2 in]
    n188 = Bundle By Name(cluster=T15 {"启动模式"=enum."跨度核查", "启动参数"=1, "量程"=enum."低量程"} ("参数簇"), "启动参数"=w211, "启动模式"=w213, "量程"=w212) -> (w205:T15)
    n189 = First Call?() -> (First Call?: T/F=w217:bool)
    n190 = case shown="真" w218 {
      tunnel: w187 -> [_ w429]
      frame False {
      }
      frame True {
        n191 = Subtract(x=w429, y=1) -> (x-y=w427:i32)
        n192 = Subtract(x=w427, y=5) -> (x-y=w431:i32)
        n193 = Greater Or Equal To 0?(x=w431) -> (x >= 0?=w430:bool)
        n194 = property on="多列列表框" class="MCListbox (严格)"() -> (error out=w435:errorcluster, "TopLeft"=w436:T18)  [unwired: 2 in, 1 out]
        n195 = Select(t=w431, s=w430, f=0) -> (s? t:f=w432:i32)
        n196 = Bundle By Name(cluster=w436, "Row"=w432) -> (w437:T18)
        n197 = property on="多列列表框" class="MCListbox (严格)"(error in=w435, "TopLeft"=w437) -> ()  [unwired: 1 in, 2 out]
      }
    }
    n198 = Or(x=w180, y=w217) -> (x .or. y?=w215:bool)
    n199 = while {
      tunnel: w215 -> [w415]
      tunnel: w205 -> [w414]
      shift-right: [w409] -> _
      shift-left: _ -> [w411]
      shift-right: [w410] -> _
      shift-left: _ -> [w412]
      stop <- TRUE stop-if-true
      n200 = case shown="真" w415 {
        tunnel: [w417 w425] -> w410
        tunnel: [w416 w424] -> w409
        tunnel: w414 -> [_ w419]
        tunnel: w412 -> [w417 _]
        tunnel: w411 -> [w416 _]
        frame False {
        }
        frame True {
          n201 = call "斯坦道XML解析.vi"("添加的路径"="流程路径", "参数簇"=w419) -> ("步骤时间"=w420:string[], "步骤名"=w422:string[])  [unwired: 8 in]
          n202 = for {
            tunnel: w422 -> [_] mode=indexing
            tunnel: [w426] -> w423 mode=indexing
            i -> [w426]
          }
          n203 = Build Array(w422, w420) -> (w421:string[][])
          n204 = Transpose 2D Array(2D array=w421) -> (transposed array=w424:string[][])
          n205 = Number To Decimal String(number=w423) -> (decimal integer string=w425:string[])  [unwired: 1 in]
        }
      }
      n206 = property on="多列列表框" class="MCListbox (严格)"("ItemNames"=w409, "RowHdrs[]"=w410) -> ()  [unwired: 2 in, 2 out]
    }
    n207 = case shown="1, 默认" w199 {
      selector: w199 -> [_ w356]
      tunnel: w202 -> [_ w357]
      tunnel: w201 -> [_ w355]
      frame 0 {
      }
      frame 1, Default {
        n208 = case shown="真" w355 {
          tunnel: w357 -> [_ w364]
          tunnel: w356 -> [_ w358]
          frame False {
          }
          frame True {
            n209 = case shown="默认" w358 {
              selector: w358 -> [w366 _ _ _ _ _ _ _ _ _ _ _ _ _ _ _ _ _ _ _ _ _ _ _ _ _ _ _ _ _ _ _ _ _ _ _ _ _]
              tunnel: [w365 "无告警" "缺试剂告警" "缺水样告警" "缺蒸馏水告警" "缺标液告警" "仪表漏液告警" "标定异常告警" "超量程告警" "加热异常" "低试剂预警" "超上限告警" "超下限告警" "仪表内部其他异常" "滴定异常告警" "电极异常告警" "量程切换告警" "参数设置告警" "PH电极电位异常" "电导率电极异常" "浊度光度异常" "溶解氧电极异常" "溶解氧光强异常" "温度异常告警" "PH异常告警" "溶解氧异常告警" "电导率异常告警" "浊度异常告警" "叶绿素异常告警" "藻密度异常告警" "蓝绿藻异常告警" "ORP异常告警" "氨氮异常告警" "清洁刷异常告警" "SD卡异常告警" "蓝牙异常告警" "WiFi异常告警" "流程异常告警"] -> w359
              frame Default {
                n210 = Format Into String(format string="%d" ("格式字符串"), initial string="内部告警-" ("工作状态"), w366) -> (resulting string=w365:string)  [unwired: 1 in, 1 out]
              }
              frame 0 {
              }
              frame 1 {
              }
              frame 2 {
              }
              frame 3 {
              }
              frame 4 {
              }
              frame 5 {
              }
              frame 6 {
              }
              frame 7 {
              }
              frame 8 {
              }
              frame 9 {
              }
              frame 10 {
              }
              frame 11 {
              }
              frame 12 {
              }
              frame 13 {
              }
              frame 14 {
              }
              frame 15 {
              }
              frame 16 {
              }
              frame 17 {
              }
              frame 18 {
              }
              frame 19 {
              }
              frame 20 {
              }
              frame 21 {
              }
              frame 22 {
              }
              frame 23 {
              }
              frame 24 {
              }
              frame 25 {
              }
              frame 26 {
              }
              frame 27 {
              }
              frame 28 {
              }
              frame 29 {
              }
              frame 30 {
              }
              frame 31 {
              }
              frame 32 {
              }
              frame 33 {
              }
              frame 34 {
              }
              frame 35 {
              }
              frame 36 {
              }
            }
            n211 = case shown="3, 92" w364 {
              tunnel: ["总磷" ("table输入") "氨氮" ("table输入") "总氮" ("table输入")] -> w360
              frame 1, 131 {
              }
              frame 3, 92 {
              }
              frame 2, 76, Default {
              }
            }
            n212 = Get Date/Time In Seconds() -> (seconds since 1Jan1904=w361:timestamp)
            n213 = Bundle By Name(cluster=T17 {"时间标识"=timestamp(0 s since 1904-01-01), "设备"="", "日志信息"=""} ("data in"), "时间标识"=w361, "设备"=w360, "日志信息"=w359) -> (w362:T17)
            n214 = call "氨氮报警信息.vi"("data in"=w362) -> ()  [unwired: 10 in, 1 out]
          }
        }
      }
    }
  }
  n215 = while {
    tunnel: w10 -> [w442]
    tunnel: [w440] -> _
    stop <- FALSE stop-if-true
    # "定时更新"
    n216 = Get Queue Status(queue=w442) -> (queue out=w439:refnum<queue>, # elements in queue=w438:i32)  [unwired: 2 in, 6 out]
    n217 = case shown="0" w438 {
      tunnel: [_ w445] -> w440
      tunnel: w439 -> [_ w444]
      frame Default {
      }
      frame 0 {
        w448 = u16 3 items=["总磷"=1, "氨氮"=3] ("站号")
        n218 = call "版本号读取.vi"() -> ("error out"=w445:errorcluster, "固件版本号"=→"固件版本号":string)  [unwired: 10 in]
        n219 = Bundle By Name(cluster=cluster{"命令":string, "data":variant} {"命令"="", "data"=variant} ("元素"), "命令"="读序列号", "data"=w448) -> (w447:cluster{"命令":string, "data":variant})
        n220 = Enqueue Element(queue=w444, element=w447) -> ()  [unwired: 2 in, 3 out]
      }
    }
    n221 = Wait (ms)(milliseconds to wait=u32 1000 ("等待时间（毫秒）")) -> ()  [unwired: 1 out]
  }
  n222 = property on="曲线模型" class="曲线模型 (严格)"("属性"=w1) -> (error out=w9:errorcluster)  [unwired: 2 in, 1 out]
  n223 = Cancel Notification(0:w6) -> (8:w5:refnum<notifier>)  [unwired: 1 in, 2 out]
  n224 = Obtain Queue(name (unnamed)="NH3N" ("名称（未命名）"), element data type=cluster{"命令":string, "data":variant} {"命令"="", "data"=variant}) -> (queue out=w20:refnum<queue>, error out=w21:errorcluster)  [unwired: 3 in, 1 out]
  n225 = while {
    tunnel: w20 -> [w456]
    tunnel: w21 -> [_]
    stop <- FALSE stop-if-true
    n226 = Get Queue Status(queue=w456) -> (queue out=w452:refnum<queue>, # elements in queue=w451:i32)  [unwired: 2 in, 6 out]
    n227 = Wait (ms)(milliseconds to wait=u32 1000 ("等待时间（毫秒）")) -> ()  [unwired: 1 out]
    n228 = global read "氨氮断电保存全局变量.vi" "流程路径"() -> (w455:path)
    n229 = case shown="0" w451 {
      tunnel: w452 -> [_ w459]
      frame Default {
      }
      frame 0 {
        w468 = u16 3 items=["总磷"=1, "氨氮"=3] ("站号")
        # "试剂填充 172 \n管路清洗108\n氨氮92\n总磷131\n总磷海水147\n总氮76\n总氮海水92"
        n230 = global read "VAR氨氮全局变量.vi" "状态告警区"() -> (w460:T4)
        n231 = Bundle By Name(cluster=cluster{"命令":string, "data":variant} {"命令"="", "data"=variant} ("元素"), "命令"="读状态告警区", "data"=w468) -> (w474:cluster{"命令":string, "data":variant})
        n232 = Bundle By Name(cluster=cluster{"命令":string, "data":variant} {"命令"="", "data"=variant} ("元素"), "命令"="读测量数据区", "data"=w468) -> (w471:cluster{"命令":string, "data":variant})
        n233 = Unbundle By Name(w460) -> ("系统时间"=w467:timestamp)
        n234 = Enqueue Element(queue=w459, element=w474) -> (queue out=w469:refnum<queue>)  [unwired: 2 in, 2 out]
        n235 = Get Date/Time In Seconds() -> (seconds since 1Jan1904=w466:timestamp)
        n236 = Subtract(x=w466, y=w467) -> (x-y=w465:dbl)
        n237 = Absolute Value(x=w465) -> (abs(x)=w464:dbl)
        n238 = Enqueue Element(queue=w469, element=w471) -> (queue out=w461:refnum<queue>)  [unwired: 2 in, 2 out]
        n239 = Greater Or Equal?(x=w464, y=120.0) -> (x >= y?=w462:bool)
        n240 = case shown="真" w462 {
          tunnel: w461 -> [_ w477]
          frame False {
          }
          frame True {
            n241 = call "氨氮启动命令.vi"("参数"=T19 {"站号"=3, "量程切换"=enum."AUTO", "控制命令"=enum."校时", "模式设置"=enum."待机", "测量间隔"=0}) -> ("启动命令"=w476:cluster{"命令":string, "data":variant})  [unwired: 10 in]
            n242 = Enqueue Element(queue=w477, element=w476) -> ()  [unwired: 2 in, 3 out]
          }
        }
      }
    }
    n243 = local write "流程路径"(w455) -> ()
    n244 = global read "氨氮断电保存全局变量.vi" "MB通信方式选择"() -> (w453:enum16{"串口", "TCP"})
    n245 = case shown="\"TCP\"" w453 {
      tunnel: [w479 w480] -> w454
      frame "串口", Default {
        n246 = global read "氨氮断电保存全局变量.vi" "VISA Resource"() -> (w479:refnum<visa-resource-name>)
      }
      frame "TCP" {
        n247 = global read "氨氮断电保存全局变量.vi" "IP"() -> (w480:string)
      }
    }
    "字符串" <- w454
  }
  n248 = control-ref of="测量模式下拉列表"() -> (w17:refnum<vi>)
  n249 = control-ref of="量程切换阈值"() -> (w15:refnum<vi>)
  n250 = control-ref of="参数下拉列表"() -> (w18:refnum<vi>)
  n251 = control-ref of="量程下拉列表"() -> (w19:refnum<vi>)
  n252 = control-ref of="备用系数"() -> (w14:refnum<vi>)
  n253 = control-ref of="公式"() -> (w16:refnum<vi>)
  n254 = while {
    tunnel: w20 -> [w488]
    tunnel: w19 -> [w487]
    tunnel: w18 -> [w486]
    tunnel: w17 -> [w485]
    tunnel: w16 -> [w484]
    tunnel: w15 -> [w483]
    tunnel: w14 -> [w482]
    tunnel: w9 -> [_]
    tunnel: w5 -> [w481]
    stop <- FALSE stop-if-true
    n255 = event shown="[7] \"曲线模型\": 值改变" {
      selector: _ -> [_ _ _ _ _ _ _ _ _ _ _ _ _ _ _ _ _ _ _ _ _ _ _ _]
      dyn-events: _ -> [_ _ _ _ _ _ _ _ _ _ _ _ _ _ _ _ _ _ _ _ _ _ _ _]
      timeout: _ -> [_ _ _ _ _ _ _ _ _ _ _ _ _ _ _ _ _ _ _ _ _ _ _ _]
      tunnel: w488 -> [_ _ w504 w532 _ _ _ _ _ _ _ w640 _ w665 w672 _ _ _ _ _ _ _ _ _]
      tunnel: w487 -> [_ _ _ _ _ _ _ _ _ _ _ _ _ _ _ _ _ _ w688 _ w722 w731 w737 w749]
      tunnel: w486 -> [_ _ _ _ _ _ _ _ _ _ _ _ _ _ _ _ _ _ w686 _ w720 w733 w745 w756]
      tunnel: w485 -> [_ _ _ _ _ _ _ _ _ _ _ _ _ _ _ _ _ _ w687 _ w721 w732 w739 w751]
      tunnel: w484 -> [_ _ _ _ _ _ _ _ _ _ _ _ _ _ _ _ _ _ w682 _ _ _ _ _]
      tunnel: w483 -> [_ _ _ _ _ _ _ _ _ _ _ _ _ _ _ _ _ _ _ _ w716 _ _ _]
      tunnel: w482 -> [_ _ _ _ _ _ _ _ _ _ _ _ _ _ _ _ _ _ _ _ _ _ w743 _]
      tunnel: w481 -> [_ _ _ _ _ _ _ _ _ _ _ _ _ _ w668 _ _ _ _ _ _ _ _ _]
      tunnel: [_ w490 _ _ _ _ _ _ _ _ _ _ _ _ _ _ _ _ _ _ _ _ _ _] -> _
      event Timeout {
        n256 = event-data() -> ()  [unwired: 1 in, 3 out]
      }
      event "测量模式下拉列表", "量程下拉列表", "参数下拉列表": Value Change {
        n257 = event-data() -> ()  [unwired: 1 in, 6 out]
        n258 = local read "参数下拉列表"() -> (w491:enum16{"总磷", "总氮", "氨氮"})
        n259 = local read "测量模式下拉列表"() -> (w492:enum16{"水样测量", "零点核查", "跨度核查", "标样核查", "加标回收"})
        n260 = local read "量程下拉列表"() -> (w493:enum16{"低量程", "高量程"})
        n261 = Bundle("参数下拉列表"=w491, "测量模式下拉列表"=w492, "量程下拉列表"=w493) -> (w494:T14)  [unwired: 1 in]
        n262 = property on="曲线模型" class="曲线模型 (严格)"("属性"=w494) -> (error out=w490:errorcluster)  [unwired: 2 in, 1 out]
      }
      event "串口设置": Value Change {
        n263 = event-data() -> ()  [unwired: 1 in, 6 out]
        n264 = global read "氨氮断电保存全局变量.vi" "MB通信方式选择"() -> (w495:enum16{"串口", "TCP"})
        n265 = global read "氨氮断电保存全局变量.vi" "VISA Resource"() -> (w501:refnum<visa-resource-name>)
        n266 = global read "氨氮断电保存全局变量.vi" "PORT"() -> (w499:string)
        n267 = global read "氨氮断电保存全局变量.vi" "IP"() -> (w500:string)
        n268 = call "串口配置.vi"("PORT"=w499, "IP"=w500, "MB通信方式选择"=w495, "请选择串口:"=w501) -> ("PORT 2"=w497:string, "IP 2"=w498:string, "确认 2"=w502:bool, "VISA资源名称 2"=w503:refnum<visa-resource-name>, "MB通信方式选择 2"=w496:enum16{"串口", "TCP"})  [unwired: 3 in]
        n269 = case shown="真" w502 {
          tunnel: w503 -> [_ w509]
          tunnel: w504 -> [_ w508]
          tunnel: w498 -> [_ w507]
          tunnel: w497 -> [_ w506]
          tunnel: w496 -> [_ w505]
          frame False {
          }
          frame True {
            n270 = flat-sequence {
              tunnel: w509 -> [w514]
              tunnel: w508 -> [w515]
              tunnel: w507 -> [w513]
              tunnel: w506 -> [w512]
              tunnel: w505 -> [w511]
              frame #0 {
                n271 = global write "氨氮断电保存全局变量.vi" "IP"(w513) -> ()
                n272 = global write "氨氮断电保存全局变量.vi" "PORT"(w512) -> ()
                n273 = global write "氨氮断电保存全局变量.vi" "VISA Resource"(w514) -> ()
                n274 = global write "氨氮断电保存全局变量.vi" "MB通信方式选择"(w511) -> ()
                n275 = Flush Queue(queue=w515) -> (queue out=w510:refnum<queue>)  [unwired: 1 in, 2 out]
                n276 = Enqueue Element(queue=w510, element=cluster{"命令":string, "data":variant} {"命令"="启用模块", "data"=variant} ("元素")) -> ()  [unwired: 2 in, 3 out]
              }
              frame #1 {
                n277 = call <vilib>:"Application Directory.vi"() -> ("Application Directory"=w530:path)
                n278 = Build Path(base path=w530, name or relative path="data\\sys.ini" ("名称或相对路径")) -> (appended path=w528:path)
                n279 = call <vilib>:"Open Config Data.vi"("configuration file path"=w528) -> ("error out"=w524:errorcluster, "refnum"=w527:T13)  [unwired: 8 in, 1 out]
                n280 = vi-ref "氨氮断电保存全局变量.vi"() -> (w526:refnum<vi>)
                n281 = call <userlib>:"Write Panel to INI__ogtk.vi"("error in (no error)"=w524, "VI ref"=w526, "refnum"=w527) -> ("error out"=w523:errorcluster, "refnum out"=w525:T13)  [unwired: 7 in]
                n282 = call <vilib>:"Close Config Data.vi"("error in (no error)"=w523, "refnum"=w525) -> ("error out"=w518:errorcluster, "file path"=w517:path)  [unwired: 8 in]
                n283 = Open/Create/Replace File(file path (use dialog)=w517, error in=w518) -> (refnum out=w521:refnum<file>, error out=w522:errorcluster)  [unwired: 4 in, 1 out]
                n284 = Flush File(refnum=w521, error in=w522) -> (refnum out=w520:refnum<file>, error out=w519:errorcluster)
                n285 = Close File(refnum=w520, error in=w519) -> ()  [unwired: 2 out]
              }
            }
          }
        }
      }
      event "模块启用": Value Change {
        n286 = event-data() -> ("OldVal"=w533:bool)  [unwired: 1 in, 5 out]
        n287 = Flush Queue(queue=w532) -> (queue out=w531:refnum<queue>)  [unwired: 1 in, 2 out]
        n288 = case shown="假" w533 {
          tunnel: w531 -> [w534 w536]
          frame False {
            n289 = Enqueue Element(queue=w534, element=cluster{"命令":string, "data":variant} {"命令"="停用模块", "data"=variant} ("元素")) -> ()  [unwired: 2 in, 3 out]
          }
          frame True {
            n290 = Enqueue Element(queue=w536, element=cluster{"命令":string, "data":variant} {"命令"="启用模块", "data"=variant} ("元素")) -> ()  [unwired: 2 in, 3 out]
          }
        }
      }
      event "流程路径": Value Change {
        n291 = event-data() -> ()  [unwired: 1 in, 6 out]
        n292 = flat-sequence {
          frame #0 {
            n293 = local read "流程路径"() -> (w538:path)
            n294 = global write "氨氮断电保存全局变量.vi" "流程路径"(w538) -> ()
          }
          frame #1 {
            n295 = call <vilib>:"Application Directory.vi"() -> ("Application Directory"=w552:path)
            n296 = Build Path(base path=w552, name or relative path="data\\sys.ini" ("名称或相对路径")) -> (appended path=w550:path)
            n297 = call <vilib>:"Open Config Data.vi"("configuration file path"=w550) -> ("error out"=w546:errorcluster, "refnum"=w549:T13)  [unwired: 8 in, 1 out]
            n298 = vi-ref "氨氮断电保存全局变量.vi"() -> (w548:refnum<vi>)
            n299 = call <userlib>:"Write Panel to INI__ogtk.vi"("error in (no error)"=w546, "VI ref"=w548, "refnum"=w549) -> ("error out"=w545:errorcluster, "refnum out"=w547:T13)  [unwired: 7 in]
            n300 = call <vilib>:"Close Config Data.vi"("error in (no error)"=w545, "refnum"=w547) -> ("error out"=w540:errorcluster, "file path"=w539:path)  [unwired: 8 in]
            n301 = Open/Create/Replace File(file path (use dialog)=w539, error in=w540) -> (refnum out=w543:refnum<file>, error out=w544:errorcluster)  [unwired: 4 in, 1 out]
            n302 = Flush File(refnum=w543, error in=w544) -> (refnum out=w542:refnum<file>, error out=w541:errorcluster)
            n303 = Close File(refnum=w542, error in=w541) -> ()  [unwired: 2 out]
          }
        }
      }
      event "公式一键写入": Value Change {
        n304 = event-data() -> ()  [unwired: 1 in, 6 out]
        n305 = local read "公式"() -> (w553:cluster{"X^2":dbl, "X":dbl, "b":dbl})
        n306 = call "公式复合写入.vi"("公式"=w553) -> ()  [unwired: 11 in]
      }
      event "备用系数一键写入": Value Change {
        n307 = event-data() -> ()  [unwired: 1 in, 6 out]
        n308 = local read "备用系数"() -> (w554:T2)
        n309 = call "量程参数复合参数写入.vi"("备用系数"=w554) -> ()  [unwired: 11 in]
      }
      event "曲线模型": Value Change {
        n310 = event-data() -> ()  [unwired: 1 in, 6 out]
        n311 = Unbundle By Name("曲线模型") -> ("X^2"=w557:dbl, "X"=w556:dbl, "B"=w555:dbl)
        n312 = local read "公式"() -> (w560:cluster{"X^2":dbl, "X":dbl, "b":dbl})
        n313 = Bundle By Name(cluster=w560, "X^2"=w557, "X"=w556, "b"=w555) -> (w559:cluster{"X^2":dbl, "X":dbl, "b":dbl})
        n314 = local write "公式"(w559) -> ()
      }
      event "质控参数设置": Value Change {
        n315 = event-data() -> ()  [unwired: 1 in, 6 out]
        n316 = global read "氨氮断电保存全局变量.vi" "质控参数设置"() -> (w561:T20)
        n317 = call "氨氮质控参数设置.vi"("质控参数设置"=w561) -> ("输出簇"=w562:T21)  [unwired: 10 in]
        n318 = Unbundle By Name(w562) -> ("确定"=w563:bool)
        n319 = case shown="真" w563 {
          tunnel: w562 -> [_ w565]
          tunnel: w561 -> [_ w564]
          frame False {
          }
          frame True {
            n320 = flat-sequence {
              tunnel: w565 -> [w572]
              tunnel: w564 -> [w571]
              frame #0 {
                n321 = Unbundle By Name(w572) -> ("跨度值"=w570:dbl, "零点标准液浓度"=w569:dbl, "跨度标准液浓度"=w568:dbl, "标准液标准浓度"=w567:dbl)
                n322 = Bundle By Name(cluster=w571, "氨氮跨度值"=w570, "氨氮零点标准液浓度"=w569, "氨氮跨度标准液浓度"=w568, "氨氮标准液标准浓度"=w567) -> (w566:T20)
                n323 = global write "氨氮断电保存全局变量.vi" "质控参数设置"(w566) -> ()
              }
              frame #1 {
                n324 = call <vilib>:"Application Directory.vi"() -> ("Application Directory"=w586:path)
                n325 = Build Path(base path=w586, name or relative path="data\\sys.ini" ("名称或相对路径")) -> (appended path=w584:path)
                n326 = call <vilib>:"Open Config Data.vi"("configuration file path"=w584) -> ("error out"=w580:errorcluster, "refnum"=w583:T13)  [unwired: 8 in, 1 out]
                n327 = vi-ref "氨氮断电保存全局变量.vi"() -> (w582:refnum<vi>)
                n328 = call <userlib>:"Write Panel to INI__ogtk.vi"("error in (no error)"=w580, "VI ref"=w582, "refnum"=w583) -> ("error out"=w579:errorcluster, "refnum out"=w581:T13)  [unwired: 7 in]
                n329 = call <vilib>:"Close Config Data.vi"("error in (no error)"=w579, "refnum"=w581) -> ("error out"=w574:errorcluster, "file path"=w573:path)  [unwired: 8 in]
                n330 = Open/Create/Replace File(file path (use dialog)=w573, error in=w574) -> (refnum out=w577:refnum<file>, error out=w578:errorcluster)  [unwired: 4 in, 1 out]
                n331 = Flush File(refnum=w577, error in=w578) -> (refnum out=w576:refnum<file>, error out=w575:errorcluster)
                n332 = Close File(refnum=w576, error in=w575) -> ()  [unwired: 2 out]
              }
            }
          }
        }
      }
      event "仪器参数设置": Value Change {
        n333 = event-data() -> ()  [unwired: 1 in, 6 out]
        n334 = global read "氨氮断电保存全局变量.vi" "氨氮仪器参数"() -> (w588:T22)
        n335 = call "仪器参数设置.vi"("氨氮仪器参数"=w588) -> ("仪器参数设置输出"=w587:T23)  [unwired: 10 in]
        n336 = Unbundle By Name(w587) -> ("确定"=w589:bool)
        n337 = case shown="真" w589 {
          tunnel: w587 -> [_ w591]
          tunnel: w588 -> [_ w590]
          frame False {
          }
          frame True {
            n338 = flat-sequence {
              tunnel: w591 -> [w608]
              tunnel: w590 -> [w607]
              frame #0 {
                n339 = Unbundle By Name(w608) -> ("测量量程"=w606:dbl, "测量精度"=w605:dbl, "测量间隔"=w604:dbl, "消解温度"=w603:dbl, "消解时长"=w601:dbl, "空白校准时间"=w600:timestamp, "曲线截距"=w599:dbl, "曲线斜率"=w598:dbl, "测量检出限"=w597:dbl, "测量信号值"=w596:dbl, "线性相关系数"=w595:dbl, "二次多项式系数"=w594:dbl, "标样校准时间"=w593:timestamp, "稀释倍数"=w592:dbl)
                n340 = Bundle By Name(cluster=w607, "测量量程"=w606, "测量精度"=w605, "测量间隔"=w604, "消解温度"=w603, "消解时长"=w601, "空白校准时间"=w600, "曲线截距"=w599, "曲线斜率"=w598, "测量检出限"=w597, "测量信号值"=w596, "线性相关系数"=w595, "二次多项式系数"=w594, "标样校准时间"=w593, "稀释倍数"=w592) -> (w602:T22)
                n341 = global write "氨氮断电保存全局变量.vi" "氨氮仪器参数"(w602) -> ()
              }
              frame #1 {
                n342 = call <vilib>:"Application Directory.vi"() -> ("Application Directory"=w622:path)
                n343 = Build Path(base path=w622, name or relative path="data\\sys.ini" ("名称或相对路径")) -> (appended path=w620:path)
                n344 = call <vilib>:"Open Config Data.vi"("configuration file path"=w620) -> ("error out"=w616:errorcluster, "refnum"=w619:T13)  [unwired: 8 in, 1 out]
                n345 = vi-ref "氨氮断电保存全局变量.vi"() -> (w618:refnum<vi>)
                n346 = call <userlib>:"Write Panel to INI__ogtk.vi"("error in (no error)"=w616, "VI ref"=w618, "refnum"=w619) -> ("error out"=w615:errorcluster, "refnum out"=w617:T13)  [unwired: 7 in]
                n347 = call <vilib>:"Close Config Data.vi"("error in (no error)"=w615, "refnum"=w617) -> ("error out"=w610:errorcluster, "file path"=w609:path)  [unwired: 8 in]
                n348 = Open/Create/Replace File(file path (use dialog)=w609, error in=w610) -> (refnum out=w613:refnum<file>, error out=w614:errorcluster)  [unwired: 4 in, 1 out]
                n349 = Flush File(refnum=w613, error in=w614) -> (refnum out=w612:refnum<file>, error out=w611:errorcluster)
                n350 = Close File(refnum=w612, error in=w611) -> ()  [unwired: 2 out]
              }
            }
          }
        }
      }
      event "自动测试量程配置": Value Change {
        n351 = event-data() -> ()  [unwired: 1 in, 6 out]
        n352 = flat-sequence {
          frame #0 {
            n353 = global write "氨氮断电保存全局变量.vi" "氨氮自动测试量程配置"("自动测试量程配置") -> ()
          }
          frame #1 {
            n354 = call <vilib>:"Application Directory.vi"() -> ("Application Directory"=w637:path)
            n355 = Build Path(base path=w637, name or relative path="data\\sys.ini" ("名称或相对路径")) -> (appended path=w635:path)
            n356 = call <vilib>:"Open Config Data.vi"("configuration file path"=w635) -> ("error out"=w631:errorcluster, "refnum"=w634:T13)  [unwired: 8 in, 1 out]
            n357 = vi-ref "氨氮断电保存全局变量.vi"() -> (w633:refnum<vi>)
            n358 = call <userlib>:"Write Panel to INI__ogtk.vi"("error in (no error)"=w631, "VI ref"=w633, "refnum"=w634) -> ("error out"=w630:errorcluster, "refnum out"=w632:T13)  [unwired: 7 in]
            n359 = call <vilib>:"Close Config Data.vi"("error in (no error)"=w630, "refnum"=w632) -> ("error out"=w625:errorcluster, "file path"=w624:path)  [unwired: 8 in]
            n360 = Open/Create/Replace File(file path (use dialog)=w624, error in=w625) -> (refnum out=w628:refnum<file>, error out=w629:errorcluster)  [unwired: 4 in, 1 out]
            n361 = Flush File(refnum=w628, error in=w629) -> (refnum out=w627:refnum<file>, error out=w626:errorcluster)
            n362 = Close File(refnum=w627, error in=w626) -> ()  [unwired: 2 out]
          }
        }
      }
      event "手动启动": Value Change {
        n363 = event-data() -> ()  [unwired: 1 in, 6 out]
        n364 = call "氨氮启动参数对话框.vi"() -> ("确认"=w638:bool, "元素"=w639:cluster{"命令":string, "data":variant})  [unwired: 10 in]
        n365 = case shown="真" w638 {
          tunnel: w640 -> [_ w642]
          tunnel: w639 -> [_ w641]
          frame False {
          }
          frame True {
            n366 = Enqueue Element(queue=w642, element=w641) -> ()  [unwired: 2 in, 3 out]
          }
        }
      }
      event "定时启动": Mouse Down {
        n367 = event-data() -> ()  [unwired: 1 in, 6 out]
        n368 = flat-sequence {
          frame #0 {
            n369 = global read "氨氮断电保存全局变量.vi" "定时控制"() -> (w644:T6)
            n370 = call "周期设置.vi"("定时控制输入"=w644) -> ("定时控制输出"=w643:T24)  [unwired: 10 in]
            n371 = global write "氨氮断电保存全局变量.vi" "定时控制"(w643) -> ()
          }
          frame #1 {
            n372 = call <vilib>:"Application Directory.vi"() -> ("Application Directory"=w658:path)
            n373 = Build Path(base path=w658, name or relative path="data\\sys.ini" ("名称或相对路径")) -> (appended path=w656:path)
            n374 = call <vilib>:"Open Config Data.vi"("configuration file path"=w656) -> ("error out"=w652:errorcluster, "refnum"=w655:T13)  [unwired: 8 in, 1 out]
            n375 = vi-ref "氨氮断电保存全局变量.vi"() -> (w654:refnum<vi>)
            n376 = call <userlib>:"Write Panel to INI__ogtk.vi"("error in (no error)"=w652, "VI ref"=w654, "refnum"=w655) -> ("error out"=w651:errorcluster, "refnum out"=w653:T13)  [unwired: 7 in]
            n377 = call <vilib>:"Close Config Data.vi"("error in (no error)"=w651, "refnum"=w653) -> ("error out"=w646:errorcluster, "file path"=w645:path)  [unwired: 8 in]
            n378 = Open/Create/Replace File(file path (use dialog)=w645, error in=w646) -> (refnum out=w649:refnum<file>, error out=w650:errorcluster)  [unwired: 4 in, 1 out]
            n379 = Flush File(refnum=w649, error in=w650) -> (refnum out=w648:refnum<file>, error out=w647:errorcluster)
            n380 = Close File(refnum=w648, error in=w647) -> ()  [unwired: 2 out]
          }
        }
      }
      event "单步测试": Value Change {
        w660 = u16 1 items=["总磷"=1, "氨氮"=3] ("站号")
        n381 = event-data() -> ()  [unwired: 1 in, 6 out]
        n382 = Bundle("站号"=w660, "总磷氨氮调试"="总磷氨氮调试") -> (w659:cluster{"站号":u16, "总磷氨氮调试":u16[]})  [unwired: 1 in]
        n383 = Bundle By Name(cluster=cluster{"命令":string, "data":variant} {"命令"="", "data"=variant} ("元素"), "命令"="debug", "data"=w659) -> (w662:cluster{"命令":string, "data":variant})
        n384 = Enqueue Element(queue=w665, element=w662) -> ()  [unwired: 2 in, 3 out]
      }
      event "停止": Value Change {
        n385 = event-data() -> ()  [unwired: 1 in, 6 out]
        n386 = Enqueue Element(queue=w672, element=cluster{"命令":string, "data":variant} {"命令"="启动", "data"=variant(cluster{"站号":u16, "控制命令输出":u16[]} {"站号"=1, "控制命令输出"=[2816]})} ("元素")) -> (queue out=w670:refnum<queue>)  [unwired: 2 in, 2 out]
        n387 = Cancel Notification(0:w668) -> (8:w669:refnum<notifier>)  [unwired: 1 in, 2 out]
        n388 = Send Notification(notification=TRUE ("通知"), notifier=w669) -> ()  [unwired: 1 in, 2 out]
        n389 = Enqueue Element(queue=w670, element=cluster{"命令":string, "data":variant} {"命令"="启动", "data"=variant(cluster{"站号":u16, "控制命令":u16[]} {"站号"=3, "控制命令"=[2816]})} ("启动命令")) -> ()  [unwired: 2 in, 3 out]
      }
      event "设置": Value Change {
        n390 = event-data() -> ()  [unwired: 1 in, 6 out]
        n391 = property on="窗格" class="Pane"("Origin"=T11 {"Horizontal"=0, "Vertical"=628} ("原点")) -> ()  [unwired: 2 in, 2 out]
      }
      event "返回": Value Change {
        n392 = event-data() -> ()  [unwired: 1 in, 6 out]
        n393 = property on="窗格" class="Pane"("Origin"=T11 {"Horizontal"=0, "Vertical"=0} ("原点")) -> ()  [unwired: 2 in, 2 out]
      }
      event "公式.X^2", "公式.X", "公式.b", "量程切换阈值.阈值", "量程切换阈值.标液浓度", "备用系数.量程上限", "备用系数.量程下限", "备用系数.检出限", "备用系数.精度": Mouse Down {
        n394 = event-data() -> ("CtlRef"=w678:refnum<vi>)  [unwired: 1 in, 5 out]
        n395 = property class="DigNum (严格)"(reference=w678) -> (reference out=w676:refnum<vi>, "Value"=w677:dbl)  [unwired: 1 in, 1 out]
        n396 = call "数字键盘.vi"("OldNumber"=w677) -> ("NewNumber"=w675:dbl)
        n397 = property class="DigNum (严格)"(reference=w676, "Val(Sgnl)"=w675) -> ()  [unwired: 1 in, 2 out]
      }
      event "读公式": Value Change {
        n398 = event-data() -> ()  [unwired: 1 in, 6 out]
        n399 = property class="Enum (严格)"(reference=w686) -> ("Value"=w685:enum16{"总磷", "总氮", "氨氮"})  [unwired: 1 in, 2 out]
        n400 = property class="Enum (严格)"(reference=w687) -> ("Value"=w684:enum16{"水样测量", "零点核查", "跨度核查", "标样核查", "加标回收"})  [unwired: 1 in, 2 out]
        n401 = property class="Enum (严格)"(reference=w688) -> ("Value"=w683:enum16{"低量程", "高量程"})  [unwired: 1 in, 2 out]
        n402 = call "公式读取.vi"("量程"=w683, "测量模式"=w684, "测量参数"=w685) -> ("error out"=w680:errorcluster, "公式"=w681:cluster{"X^2":dbl, "X":dbl, "b":dbl})  [unwired: 7 in]
        n403 = property class="Clust (严格)"(reference=w682, "Value"=w681) -> ()  [unwired: 1 in, 2 out]
        n404 = case shown="错误" w680 {
          tunnel: ["读取成功" ("消息") "读取失败" ("消息")] -> w679
          frame No Error {
          }
          frame Error {
          }
        }
        n405 = One Button Dialog(message=w679) -> ()  [unwired: 1 in, 1 out]
      }
      event "写公式": Value Change {
        n406 = event-data() -> ()  [unwired: 1 in, 6 out]
        n407 = call "公式写入.vi"("公式"="公式", "量程"="量程下拉列表", "测量模式"="测量模式下拉列表", "测量参数"="参数下拉列表") -> ("error out"=w695:errorcluster)  [unwired: 7 in]
        n408 = case shown="无错误" w695 {
          tunnel: ["写入成功" ("消息") "写入失败" ("消息")] -> w696
          tunnel: "测量模式下拉列表" -> [w702 _]
          tunnel: "量程下拉列表" -> [w701 _]
          tunnel: "公式" -> [w697 _]
          frame No Error {
            n409 = Equal?(x=w702, y=enum16{"水样测量", "零点核查", "跨度核查", "标样核查", "加标回收"}."水样测量") -> (x = y?=w700:bool)
            n410 = Equal?(x=w701, y=enum16{"低量程", "高量程"}."低量程") -> (x = y?=w699:bool)
            n411 = And(x=w700, y=w699) -> (x .and. y?=w698:bool)
            n412 = case shown="真" w698 {
              tunnel: w697 -> [_ w706]
              frame False {
              }
              frame True {
                n413 = Unbundle By Name(w706) -> ("X^2"=w709:dbl, "X"=w708:dbl, "b"=w707:dbl)
                n414 = global read "氨氮断电保存全局变量.vi" "氨氮仪器参数"() -> (w710:T22)
                n415 = Bundle By Name(cluster=w710, "曲线截距"=w707, "曲线斜率"=w708, "二次多项式系数"=w709) -> (w711:T22)
                n416 = global write "氨氮断电保存全局变量.vi" "氨氮仪器参数"(w711) -> ()
              }
            }
          }
          frame Error {
          }
        }
        n417 = One Button Dialog(message=w696) -> ()  [unwired: 1 in, 1 out]
      }
      event "量程切换阈值读取": Value Change {
        n418 = event-data() -> ()  [unwired: 1 in, 6 out]
        n419 = property class="Enum (严格)"(reference=w720) -> ("Value"=w719:enum16{"总磷", "总氮", "氨氮"})  [unwired: 1 in, 2 out]
        n420 = property class="Enum (严格)"(reference=w721) -> ("Value"=w718:enum16{"水样测量", "零点核查", "跨度核查", "标样核查", "加标回收"})  [unwired: 1 in, 2 out]
        n421 = property class="Enum (严格)"(reference=w722) -> ("Value"=w717:enum16{"低量程", "高量程"})  [unwired: 1 in, 2 out]
        n422 = call "量程读取.vi"("量程"=w717, "测量模式"=w718, "测量参数"=w719) -> ("error out"=w713:errorcluster, "量程切换阈值"=w715:cluster{"阈值":dbl, "标液浓度":dbl})  [unwired: 7 in]
        n423 = property class="Clust (严格)"(reference=w716, "Value"=w715) -> ()  [unwired: 1 in, 2 out]
        n424 = case shown="错误" w713 {
          tunnel: ["读取成功" ("消息") "读取失败" ("消息")] -> w714
          frame No Error {
          }
          frame Error {
          }
        }
        n425 = One Button Dialog(message=w714) -> ()  [unwired: 1 in, 1 out]
      }
      event "量程切换阈值写入": Value Change {
        n426 = event-data() -> ()  [unwired: 1 in, 6 out]
        n427 = property class="Enum (严格)"(reference=w733) -> ("Value"=w730:enum16{"总磷", "总氮", "氨氮"})  [unwired: 1 in, 2 out]
        n428 = property class="Enum (严格)"(reference=w732) -> ("Value"=w729:enum16{"水样测量", "零点核查", "跨度核查", "标样核查", "加标回收"})  [unwired: 1 in, 2 out]
        n429 = property class="Enum (严格)"(reference=w731) -> ("Value"=w728:enum16{"低量程", "高量程"})  [unwired: 1 in, 2 out]
        n430 = call "量程写入.vi"("量程切换阈值"="量程切换阈值", "量程"=w728, "测量模式"=w729, "测量参数"=w730) -> ("error out"=w725:errorcluster)  [unwired: 7 in]
        n431 = case shown="无错误" w725 {
          tunnel: ["写入成功" ("消息") "写入失败" ("消息")] -> w726
          frame No Error {
          }
          frame Error {
          }
        }
        n432 = One Button Dialog(message=w726) -> ()  [unwired: 1 in, 1 out]
      }
      event "备用系数读取": Value Change {
        n433 = event-data() -> ()  [unwired: 1 in, 6 out]
        n434 = property class="Enum (严格)"(reference=w745) -> ("Value"=w744:enum16{"总磷", "总氮", "氨氮"})  [unwired: 1 in, 2 out]
        n435 = property class="Enum (严格)"(reference=w739) -> ("Value"=w738:enum16{"水样测量", "零点核查", "跨度核查", "标样核查", "加标回收"})  [unwired: 1 in, 2 out]
        n436 = property class="Enum (严格)"(reference=w737) -> ("Value"=w736:enum16{"低量程", "高量程"})  [unwired: 1 in, 2 out]
        n437 = call "备用系数读取.vi"("量程"=w736, "测量模式"=w738, "测量参数"=w744) -> ("error out"=w740:errorcluster, "备用系数"=w742:T2)  [unwired: 7 in]
        n438 = property class="Clust (严格)"(reference=w743, "Value"=w742) -> ()  [unwired: 1 in, 2 out]
        n439 = case shown="错误" w740 {
          tunnel: ["读取成功" ("消息") "读取失败" ("消息")] -> w741
          frame No Error {
          }
          frame Error {
          }
        }
        n440 = One Button Dialog(message=w741) -> ()  [unwired: 1 in, 1 out]
      }
      event "备用系数写入": Value Change {
        n441 = event-data() -> ()  [unwired: 1 in, 6 out]
        n442 = property class="Enum (严格)"(reference=w756) -> ("Value"=w755:enum16{"总磷", "总氮", "氨氮"})  [unwired: 1 in, 2 out]
        n443 = property class="Enum (严格)"(reference=w751) -> ("Value"=w750:enum16{"水样测量", "零点核查", "跨度核查", "标样核查", "加标回收"})  [unwired: 1 in, 2 out]
        n444 = property class="Enum (严格)"(reference=w749) -> ("Value"=w748:enum16{"低量程", "高量程"})  [unwired: 1 in, 2 out]
        n445 = call "备用系数写入.vi"("备用系数"="备用系数", "量程"=w748, "测量模式"=w750, "测量参数"=w755) -> ("error out"=w752:errorcluster)  [unwired: 7 in]
        n446 = case shown="无错误" w752 {
          tunnel: ["写入成功" ("消息") "写入失败" ("消息")] -> w753
          frame No Error {
          }
          frame Error {
          }
        }
        n447 = One Button Dialog(message=w753) -> ()  [unwired: 1 in, 1 out]
      }
    }
  }
